vi "Intake Teleop Handler.vi"() -> ()   [LabVIEW 2025]
uses:
  <vilib>/Rock Robotics/WPI/Joystick/XBox Axes Indexer.ctl
  <vilib>/Rock Robotics/WPI/Joystick/XBox Buttons Indexer.ctl
  Intake/Implementation/Intake Operations.ctl
  Pivot/Implementation/Pivot Operations.ctl
  <vilib>/Rock Robotics/WPI/Utilities/WPI_GetSetVariantRefNum.vi
  Globals.vi
panel:
  in  "Roller Speed Outtake":dbl=0.4 format="%#_13g"
  in  "Roller Speed":dbl=-0.8 format="%#_13g"
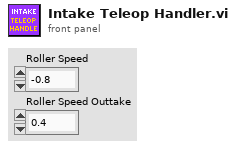
[diagram p1: front panel]
types:
  T1 = typedef "XBox Buttons Indexer.ctl" = enum16{"A", "B", "X", "Y", "Left Bumper", "Right Bumper", "Back", "Start", "Left Joystick", "Right Joystick"}
  T2 = typedef "XBox Axes Indexer.ctl" = enum16{"Left X", "Left Y", "Left Trigger", "Right Trigger", "Right X", "Right Y"}
  T3 = typedef "WPI_JoystickDevRef.ctl" = cluster{"Device":T4}
  T4 = typedef "WPI_JoystickDeviceEnum.ctl" = enum16{"USB 0", "USB 1", "USB 2", "USB 3", "USB 4", "USB 5"}
  T5 = typedef "Intake Operations.ctl" = enum16{"Reserve", "Read Current", "Immediate", ""}
  T6 = typedef "Pivot Operations.ctl" = enum16{"Reserve", "Read Current", "Retract Pivot", "Extend Pivot", "Reset Pivot", "Immediate"}
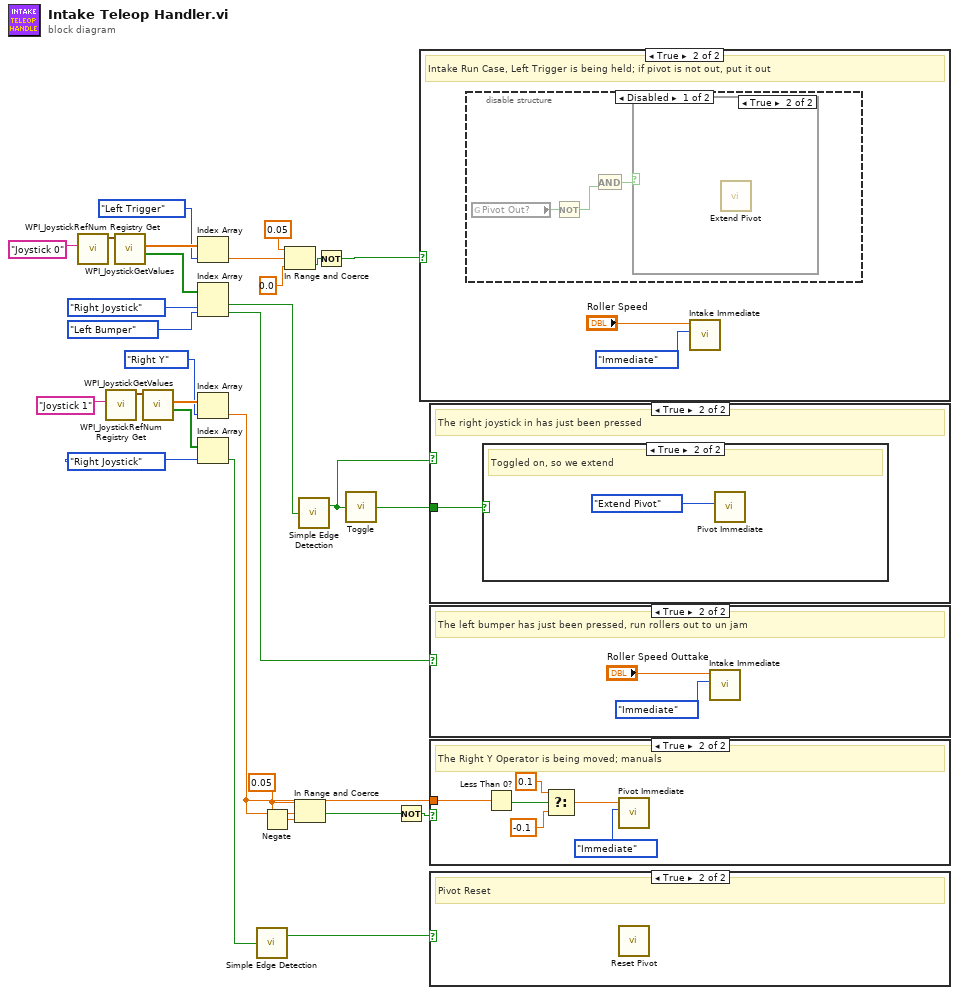
[diagram p0: block diagram]
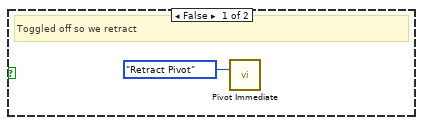
[diagram p5: hidden frame]
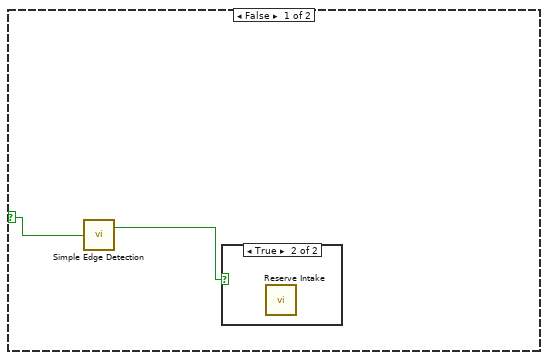
[diagram p7: hidden frame]
diagram:
  w11 = 0.05 ("upper limit")
  n1 = call <vilib>:"WPI_JoystickRefNum Registry Get.vi"("refnum name"="Joystick 0") -> ("JoystickDevRef"=w28:T3)  [unwired: 1 in, 9 out]
  n2 = call <vilib>:"WPI_JoystickRefNum Registry Get.vi"("refnum name"="Joystick 1") -> ("JoystickDevRef"=w23:T3)  [unwired: 1 in, 9 out]
  n3 = call <vilib>:"WPI_JoystickGetValues.vi"("JoystickDevRef"=w28) -> ("Buttons"=w25:bool[], "Axes"=w27:dbl[])  [unwired: 6 in, 3 out]
  n4 = call <vilib>:"WPI_JoystickGetValues.vi"("JoystickDevRef"=w23) -> ("Buttons"=w19:bool[], "Axes"=w22:dbl[])  [unwired: 6 in, 3 out]
  n5 = Index Array(array=w27, index=XBox_Axes_Indexer."Left Trigger" ("XBox Axes")) -> (element=w15:dbl)
  n6 = Index Array(array=w25, index #1=XBox_Buttons_Indexer."Right Joystick" ("XBox Buttons"), index #2=XBox_Buttons_Indexer."Left Bumper" ("XBox Buttons")) -> (element #1=w13:bool, element #2=w1:bool)
  n7 = Index Array(array=w22, index=XBox_Axes_Indexer."Right Y" ("XBox Axes")) -> (element=w10:dbl)
  n8 = Index Array(array=w19, index=XBox_Buttons_Indexer."Right Joystick" ("XBox Buttons")) -> (element=w7:bool)
  n9 = call "Simple Edge Detection.vi"("In"=w7) -> ("Rising Edge"=w6:bool)  [unwired: 1 out]
  n10 = Negate(x=w11) -> (-x=w12:dbl)
  n11 = In Range and Coerce(upper limit=0.05, x=w15, lower limit=0.0) -> (In Range?=w14:bool)  [unwired: 1 out]
  n12 = In Range and Coerce(upper limit=w11, x=w10, lower limit=w12) -> (In Range?=w9:bool)  [unwired: 1 out]
  n13 = call "Simple Edge Detection.vi"("In"=w13) -> ("Rising Edge"=w4:bool)  [unwired: 1 out]
  n14 = Not(x=w14) -> (.not. x?=w5:bool)
  n15 = call "Toggle.vi"("In"=w4) -> ("Toggled Output"=w3:bool)
  n16 = Not(x=w9) -> (.not. x?=w8:bool)
  n17 = case shown="True" w5 {
    selector: w5 -> [w31 _]
    frame False {
      n18 = call "Simple Edge Detection.vi"("In"=w31) -> ("Rising Edge"=w30:bool)  [unwired: 1 out]
      n19 = case shown="True" w30 {
        frame False {
        }
        frame True {
          n20 = call "Reserve Intake.vi"() -> ()  [unwired: 11 in, 1 out]
        }
      }
    }
    frame True {
      # "Intake Run Case, Left Trigger is being held; if pivot is not out, put it out"
      n21 = disable-structure shown="Disabled" {
        frame Disabled {
          n22 = global read "Globals.vi" "Pivot Out?"() -> (w36:bool)
          n23 = Not(x=w36) -> (.not. x?=w34:bool)
          n24 = And(y=w34) -> (x .and. y?=w35:bool)  [unwired: 1 in]
          n25 = case shown="True" w35 {
            frame False {
            }
            frame True {
              n26 = call "Extend Pivot.vi"() -> ()  [unwired: 11 in, 1 out]
            }
          }
        }
        frame Enabled {
        }
      }
      n27 = call "Intake Immediate.vi"("Operation"=Intake_Operations."Immediate", "Setpoint"="Roller Speed") -> ()  [unwired: 9 in, 1 out]
    }
  }
  n28 = case shown="True" w4 {
    tunnel: w3 -> [_ w37]
    frame False {
    }
    frame True {
      # "The right joystick in has just been pressed"
      n29 = case shown="True" w37 {
        frame False {
          # "Toggled off so we retract"
          n30 = call "Pivot Immediate.vi"("Operation"=Pivot_Operations."Retract Pivot") -> ()  [unwired: 10 in, 1 out]
        }
        frame True {
          # "Toggled on, so we extend"
          n31 = call "Pivot Immediate.vi"("Operation"=Pivot_Operations."Extend Pivot") -> ()  [unwired: 10 in, 1 out]
        }
      }
    }
  }
  n32 = case shown="True" w1 {
    frame False {
    }
    frame True {
      # "The left bumper has just been pressed, run rollers out to un jam"
      n33 = call "Intake Immediate.vi"("Operation"=Intake_Operations."Immediate", "Setpoint"="Roller Speed Outtake") -> ()  [unwired: 9 in, 1 out]
    }
  }
  n34 = case shown="True" w8 {
    tunnel: w10 -> [_ w47]
    frame False {
    }
    frame True {
      # "The Right Y Operator is being moved; manuals"
      n35 = Less Than 0?(x=w47) -> (x < 0?=w46:bool)
      n36 = Select(t=0.1, s=w46, f=-0.1 ("t")) -> (s? t:f=w43:dbl)
      n37 = call "Pivot Immediate.vi"("Operation"=Pivot_Operations."Immediate", "Setpoint"=w43) -> ()  [unwired: 9 in, 1 out]
    }
  }
  n38 = case shown="True" w6 {
    frame False {
    }
    frame True {
      # "Pivot Reset"
      n39 = call "Reset Pivot.vi"() -> ()  [unwired: 11 in, 1 out]
    }
  }
